vi "测试.vi"   [LabVIEW 2012]
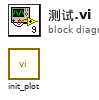
[diagram p0: block diagram]
diagram:
  n1 = call "init_plot.vi"() -> ()  [unwired: 4 in, 2 out]
